vi "AskForConnectedMonos.vi"(7 "DiscoverDevices in":T1, 8 "error in (no error)":errorcluster, 10 "timeout for receiving data [ms]":i32=5000, 11 "Communicator in":refnum<class "Communicator.lvclass">) -> (0 "error out":errorcluster, 2 "DiscoverDevices out":T1, 3 "Communicator out":refnum<class "Communicator.lvclass">)   [LabVIEW 2023, in "DeviceManager.lvlib"]
uses:
  DeviceManager.lvlib
  DiscoverDevices (Reply Payload)--cluster.ctl
  Classes/Mono/Monochromator.lvclass
  Classes/CCD/CCD.lvclass
  Classes/SCD/SCD.lvclass
  Classes/Communicator/Communicator.lvclass
  Classes/GenericDevice/GenericDevice.lvclass
panel:
  # "Connector Pane"
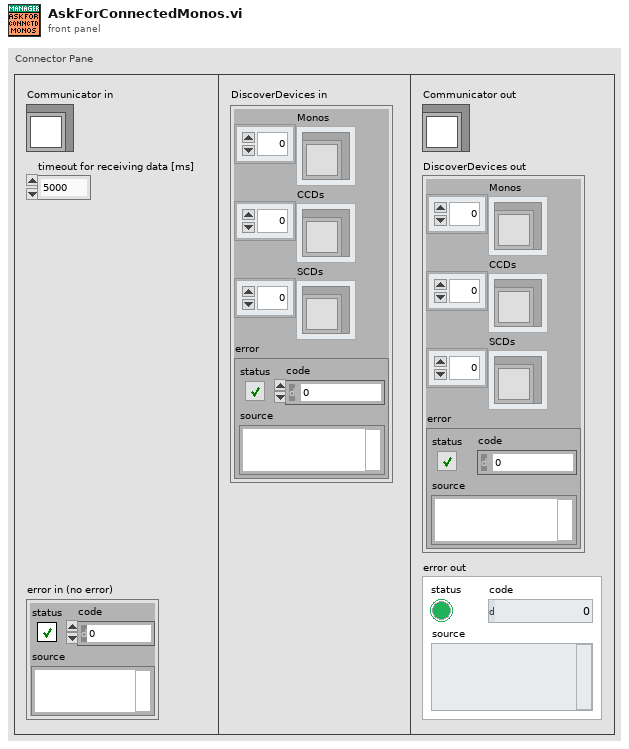
[diagram p1: front panel]
types:
  T1 = typedef "DeviceManager.lvlib/DiscoverDevices (Reply Payload)--cluster.ctl" = cluster{"Monos":refnum<class "Monochromator.lvclass">[], "CCDs":refnum<class "CCD.lvclass">[], "SCDs":refnum<class "SCD.lvclass">[], "error":errorcluster}
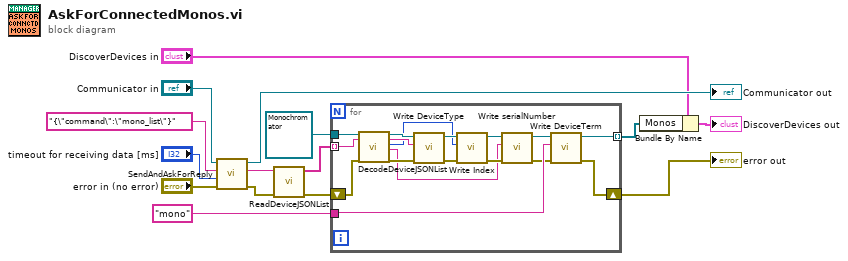
[diagram p0: block diagram]
diagram:
  n1 = call-dynamic "SendAndAskForReply.vi"("error in (no error)"="error in (no error)", "timeout for receiving data [ms]"="timeout for receiving data [ms]", "String to be sent"="{\"command\":\"mono_list\"}", "Communicator in"="Communicator in") -> ("error out"=w6:errorcluster, "Data"=w5:string, "Communicator out"=→"Communicator out":refnum<class "Communicator.lvclass">)  [unwired: 5 in]
  n2 = call "ReadDeviceJSONList.vi"("error in"=w6, "JSON"=w5) -> ("error out"=w3:errorcluster, "table of devices"=w4:string[])  [unwired: 8 in]
  n3 = for {
    tunnel: w4 -> [w23] mode=indexing
    shift-right: [w16] -> w7
    shift-left: w3 -> [w21]
    tunnel: refnum<class "Monochromator.lvclass"> refnum ("Monochromator.lvclass") -> [w22]
    tunnel: [w18] -> w2 mode=indexing
    tunnel: "mono" -> [w20]
    n4 = call "DecodeDeviceJSONList.vi"("GenericDevice in"=w22, "JSON"=w23, "error in"=w21) -> ("GenericDevice out"=w32:refnum<class "Monochromator.lvclass">, "deviceType"=w26:string, "index"=w25:i32, "serialNumber"=w24:string, "error out"=w30:errorcluster)  [unwired: 11 in, 1 out]
    n5 = call-dynamic "Write DeviceType.vi"("error in (no error)"=w30, "device type"=w26, "Monochromator in"=w32) -> ("error out"=w29:errorcluster, "Monochromator out"=w31:refnum<class "Monochromator.lvclass">)  [unwired: 7 in]
    n6 = call-dynamic "Write Index.vi"("error in (no error)"=w29, "Index"=w25, "Monochromator in"=w31) -> ("error out"=w28:errorcluster, "Monochromator out"=w27:refnum<class "Monochromator.lvclass">)  [unwired: 7 in]
    n7 = call-dynamic "Write serialNumber.vi"("error in (no error)"=w28, "serialNumber"=w24, "Monochromator in"=w27) -> ("error out"=w17:errorcluster, "Monochromator out"=w19:refnum<class "Monochromator.lvclass">)  [unwired: 7 in]
    n8 = call-dynamic "Write DeviceTerm.vi"("error in (no error)"=w17, "deviceTerm"=w20, "Monochromator in"=w19) -> ("error out"=w16:errorcluster, "Monochromator out"=w18:refnum<class "Monochromator.lvclass">)  [unwired: 7 in]
  }
  "error out" <- w7
  n9 = Bundle By Name(cluster="DiscoverDevices in", "Monos"=w2) -> (→"DiscoverDevices out":T1)
